vi "Pickering 4 wire _Patrick.vi"(8 "error in (no error)":errorcluster, 11 "Y Channels":string[][](array[combo])=[["NC", "NC"], ["y1", "NC"], ["y2", ""], ["y4", ""], ["NC", ""], ["y5", ""], ["y8", ""], ["y3", ""], ["NC", ""], ["y7", ""], ["y6", ""]]) -> (0 "error out":errorcluster)   [LabVIEW 2016, in "pickering.lvclass"]
uses:
  pickering.lvclass
  Typedefs/Channels-Array.ctl
  Typedefs/Channel-Cluster.ctl
  Typedefs/ChannelX-ComboBox.ctl
  Typedefs/ChannelY-ComboBox.ctl
panel:
  in  "Tab Control":enum32{"Crosspoint Selection", "Setup"}(tab)
  in  "X Channels":string[](array[combo])=["x1", "x2", "x3", "x4", "x5", "x6", "x7", "x8", "x9", "x10", "x11"]
  in  "Pickering status":path=path "C:/Local_LabVIEW/New Text Document.txt"
  in  "VISA Resource Name":string="PXI13::13::INSTR"
  in  "Initialize":bool
  in  "Disconnect all?":bool
  in  "Discharge X channels?":bool=TRUE
  in  "Discharge Y Channels?":bool=TRUE
  in  "Y Channel Ground":string="y1"
  in  "X Channel Ground":string="x12"
  in  "IVI Option String":string="Simulate=0,RangeCheck=1,QueryInstrStatus=0,Cache=1,DriverSetup=Model:40-726-511-M;"
  # "Lock-in 1: I+/I- -->AO0/AI0, board 0\n\nLock-in 3: V+/V-  --> AI0, board 1.  \n  V+/V- conencted to y3 and y4. OSC output should set the same as Lock-in 1\n\nLock-in 2: I2+/I2- -->AO1/AI1, board 0\n\nLock-in 4: V2+/V2- -> y7/y8"
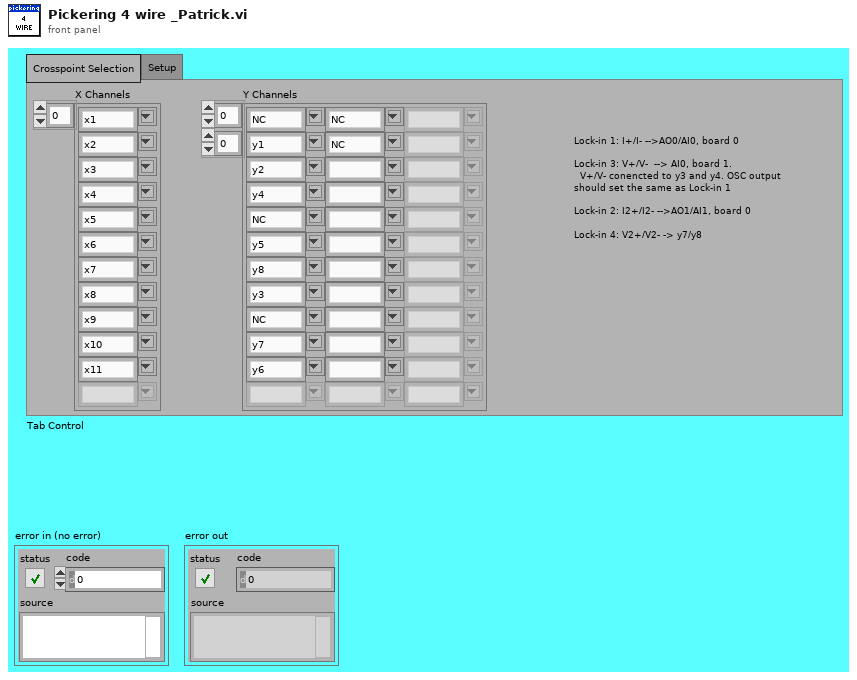
[diagram p1: front panel]
types:
  T1 = typedef "pickering.lvclass/Channels-Array.ctl" = T2[]
  T2 = typedef "pickering.lvclass/Channel-Cluster.ctl" = cluster{"Channel x":T3, "Channel y":T4}
  T3 = typedef "pickering.lvclass/ChannelX-ComboBox.ctl" = string
  T4 = typedef "pickering.lvclass/ChannelY-ComboBox.ctl" = string
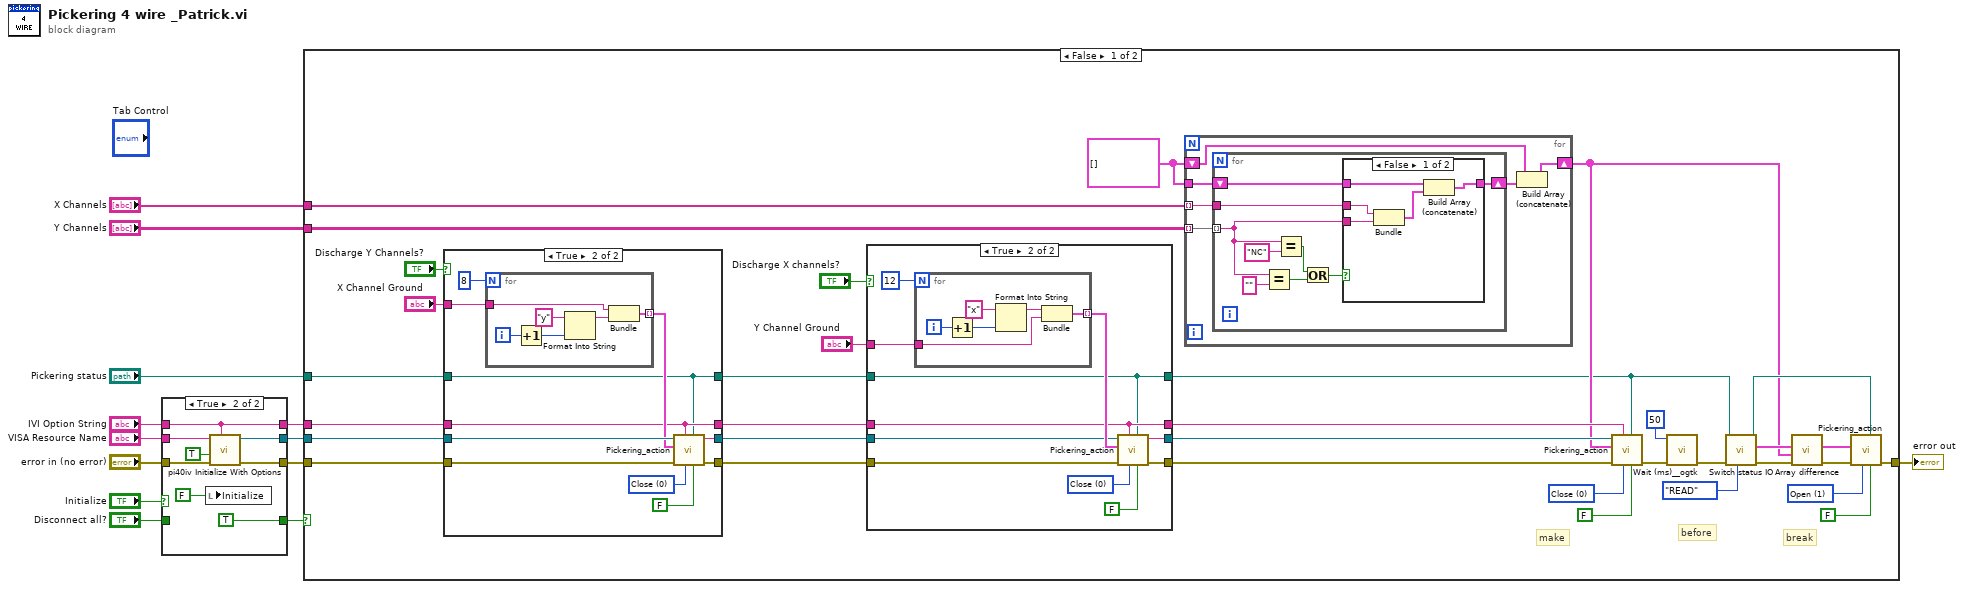
[diagram p0: block diagram]
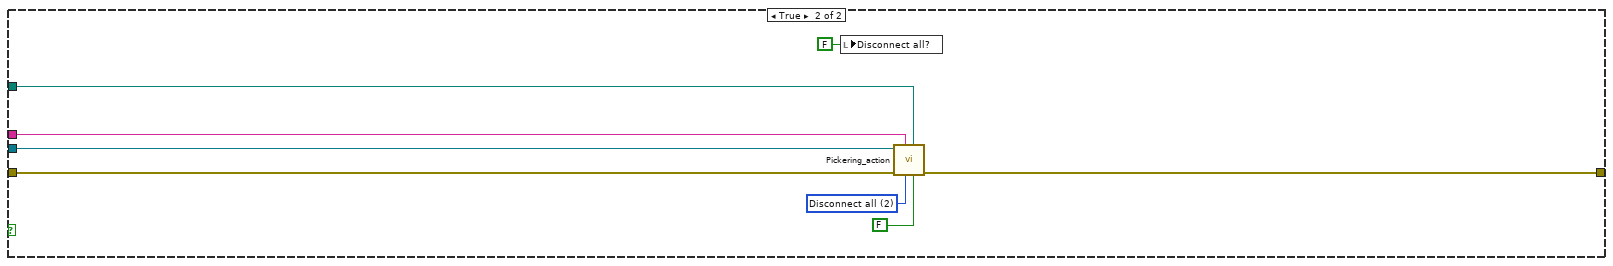
[diagram p5: hidden frame]
diagram:
  n1 = case shown="True" "Initialize" {
    tunnel: "VISA Resource Name" -> [w17 w25]
    tunnel: [w17 w21] -> w4
    tunnel: "IVI Option String" -> [w16 w24]
    tunnel: [w16 w24] -> w9
    tunnel: "Disconnect all?" -> [w15 _]
    tunnel: [w15 TRUE ("reset device")] -> w6
    tunnel: [w14 w20] -> w3
    tunnel: "error in (no error)" -> [w14 w18]
    frame False {
    }
    frame True {
      n2 = local write "Initialize"(FALSE ("reset device")) -> ()
      n3 = call <instrlib>:"pi40iv Initialize With Options.vi"("option string"=w24, "error in (no error)"=w18, "reset device"=TRUE, "resource name"=w25) -> ("error out"=w20:errorcluster, "instrument handle out"=w21:refnum<k15>)  [unwired: 6 in]
    }
  }
  n4 = case shown="False" w6 {
    tunnel: "Y Channels" -> [w50 _]
    tunnel: "X Channels" -> [w46 _]
    tunnel: w9 -> [w59 w127]
    tunnel: w4 -> [w58 w129]
    tunnel: "Pickering status" -> [w57 w125]
    tunnel: w3 -> [w56 w128]
    tunnel: [w55 w123] -> w1
    frame False {
      w32 = u16 1 items=["Close", "Open", "Disconnect all"] ("Action")
      w39 = u16 0 items=["Close", "Open", "Disconnect all"] ("Action")
      w27 = T1 []
      # "break"
      # "before"
      # "make"
      n5 = case shown="True" "Discharge Y Channels?" {
        tunnel: "X Channel Ground" -> [_ w74]
        tunnel: w59 -> [w61 w65]
        tunnel: w58 -> [w63 w72]
        tunnel: w57 -> [w60 w64]
        tunnel: w56 -> [w62 w68]
        tunnel: [w62 w67] -> w51
        tunnel: [w63 w66] -> w53
        tunnel: [w61 w65] -> w54
        tunnel: [w60 w64] -> w52
        frame False {
        }
        frame True {
          w69 = u16 0 items=["Close", "Open", "Disconnect all"] ("Action")
          n6 = for {
            N: 8 -> [_]
            tunnel: w74 -> [w76]
            tunnel: [w75] -> w71 mode=indexing
            i -> [w79]
            n7 = Increment(x=w79) -> (x+1=w78:i32)
            n8 = Format Into String(initial string="y", w78) -> (resulting string=w77:string)  [unwired: 2 in, 1 out]
            n9 = Bundle("X Channel Ground"=w76, w77) -> (w75:cluster{"X Channel Ground":string, string})  [unwired: 1 in]
          }
          n10 = call "Pickering_action.vi"("Initialize"=FALSE, "Pickering status"=w64, "Action"=w69, "option string"=w65, "error in (no error)"=w68, "Channels Array"=w71, "instrument handle"=w72) -> ("error out"=w67:errorcluster, "instrument handle out"=w66:string)  [unwired: 3 in]
        }
      }
      n11 = case shown="True" "Discharge X channels?" {
        tunnel: "Y Channel Ground" -> [_ w116]
        tunnel: w52 -> [w102 w106]
        tunnel: w53 -> [w104 w113]
        tunnel: w54 -> [w105 w109]
        tunnel: w51 -> [w103 w110]
        tunnel: [w105 w109] -> w49
        tunnel: [w103 w108] -> w47
        tunnel: [w104 w107] -> w48
        tunnel: [w102 w106] -> w26
        frame False {
        }
        frame True {
          w111 = u16 0 items=["Close", "Open", "Disconnect all"] ("Action")
          n12 = for {
            N: 12 -> [_]
            tunnel: w116 -> [w117]
            tunnel: [w119] -> w114 mode=indexing
            i -> [w121]
            n13 = Increment(x=w121) -> (x+1=w120:i32)
            n14 = Format Into String(initial string="x", w120) -> (resulting string=w118:string)  [unwired: 2 in, 1 out]
            n15 = Bundle(w118, "Y Channel Ground"=w117) -> (w119:cluster{string, "Y Channel Ground":string})  [unwired: 1 in]
          }
          n16 = call "Pickering_action.vi"("Initialize"=FALSE, "Pickering status"=w106, "Action"=w111, "option string"=w109, "error in (no error)"=w110, "Channels Array"=w114, "instrument handle"=w113) -> ("error out"=w108:errorcluster, "instrument handle out"=w107:string)  [unwired: 3 in]
        }
      }
      n17 = for {
        tunnel: w50 -> [w85] mode=indexing
        tunnel: w46 -> [w86] mode=indexing
        shift-right: [w81] -> w28
        shift-left: w27 -> [w83]
        tunnel: w27 -> [w82]
        n18 = for {
          tunnel: w86 -> [w90]
          tunnel: w85 -> [w89] mode=indexing
          shift-right: [w88] -> w84
          shift-left: w82 -> [w87]
          n19 = Equal?(x=w89, y="") -> (x = y?=w92:bool)
          n20 = Equal?(x=w89, y="NC") -> (x = y?=w94:bool)
          n21 = Or(x=w94, y=w92) -> (x .or. y?=w93:bool)
          n22 = case shown="False" w93 {
            tunnel: w90 -> [w96 _]
            tunnel: w89 -> [w97 _]
            tunnel: [w99 w101] -> w88
            tunnel: w87 -> [w98 w101]
            frame False {
              n23 = Bundle("Channel x"=w96, "Channel y"=w97) -> (w100:cluster{"Channel x":string, "Channel y":string})  [unwired: 1 in]
              n24 = Build Array (concatenate)(w98, w100) -> (w99:T1)
            }
            frame True {
            }
          }
        }
        n25 = Build Array (concatenate)(w83, w84) -> (w81:T1)
      }
      n26 = call "Pickering_action.vi"("Initialize"=FALSE, "Pickering status"=w26, "Action"=w39, "option string"=w49, "error in (no error)"=w47, "Channels Array"=w28, "instrument handle"=w48) -> ("error out"=w34:errorcluster)  [unwired: 3 in, 1 out]
      n27 = call <userlib>:"Wait (ms)__ogtk.vi"("error in (no error)"=w34, "milliseconds to wait"=u32 50) -> ("error out"=w36:errorcluster)  [unwired: 8 in, 1 out]
      n28 = call "Switch status IO.vi"("mode"=enum16{"READ", "WRITE"}."READ", "error in (no error)"=w36, "Path"=w26) -> ("error out"=w30:errorcluster, "Channels out"=w35:T1, "Path out"=w33:path)  [unwired: 6 in]
      n29 = call "Array difference.vi"("error in (no error)"=w30, "Channels Array 2"=w28, "Channels Array"=w35) -> ("error out"=w31:errorcluster, "Array 1-(array1&2)"=w41:T1)  [unwired: 6 in, 1 out]
      n30 = call "Pickering_action.vi"("Initialize"=FALSE, "Pickering status"=w33, "Action"=w32, "error in (no error)"=w31, "Channels Array"=w41) -> ("error out"=w55:errorcluster)  [unwired: 5 in, 1 out]
    }
    frame True {
      w126 = u16 2 items=["Close", "Open", "Disconnect all"] ("Action")
      n31 = local write "Disconnect all?"(FALSE ("Disconnect all?")) -> ()
      n32 = call "Pickering_action.vi"("Initialize"=FALSE, "Pickering status"=w125, "Action"=w126, "option string"=w127, "error in (no error)"=w128, "instrument handle"=w129) -> ("error out"=w123:errorcluster)  [unwired: 4 in, 1 out]
    }
  }
  "error out" <- w1
